vi "Get Controls.vi"(8 "error in (no error)":errorcluster, 10 "Root Ref":refnum<vi>, 11 "Element Filter in":refnum<class "Element Filter.lvclass">) -> (0 "error out":errorcluster, 2 "Controls":refnum<class "Control.lvclass">[](array[class]), 3 "Element Filter out":refnum<class "Element Filter.lvclass">)   [LabVIEW 2020, in "Aether Engine.lvlib" / "Element Filter.lvclass"]
uses:
  Element Filter.lvclass
  Control/Control.lvclass
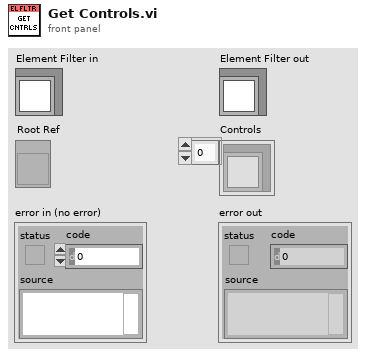
[diagram p1: front panel]
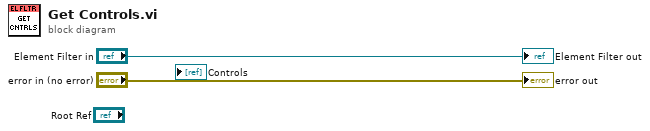
[diagram p0: block diagram]
diagram:
  "error out" <- "error in (no error)"
  "Element Filter out" <- "Element Filter in"
